vi "Signal property(SubVI).vi"(0 "Channel A":dbl[](array[numeric]), 1 "Analyze Channel":u16, 2 "DC level CH A":dbl, 3 "DC level CH B":dbl, 5 "Channel B":dbl[](array[numeric]), 7 "Channel A(FFT)":dbl[](array[numeric]), 9 "Channel B(FFT)":dbl[](array[numeric]), 11 "Frequency axis":dbl[](array[numeric]), 12 "Tones":enum32{"Single Tone", "Double tone", "Other"}(ring), 13 "Mark Signal Props":bool, 14 "Mark Harmonics":bool) -> (4 "Signal Property":string, 15 "Mark Signal Props":dbl[](array[numeric]))   [LabVIEW 2013]
uses:
  <vilib>/measure/matone.llb/SINAD Analyzer 1 Chan.vi
  <vilib>/measure/NI_MAPro.lvlib
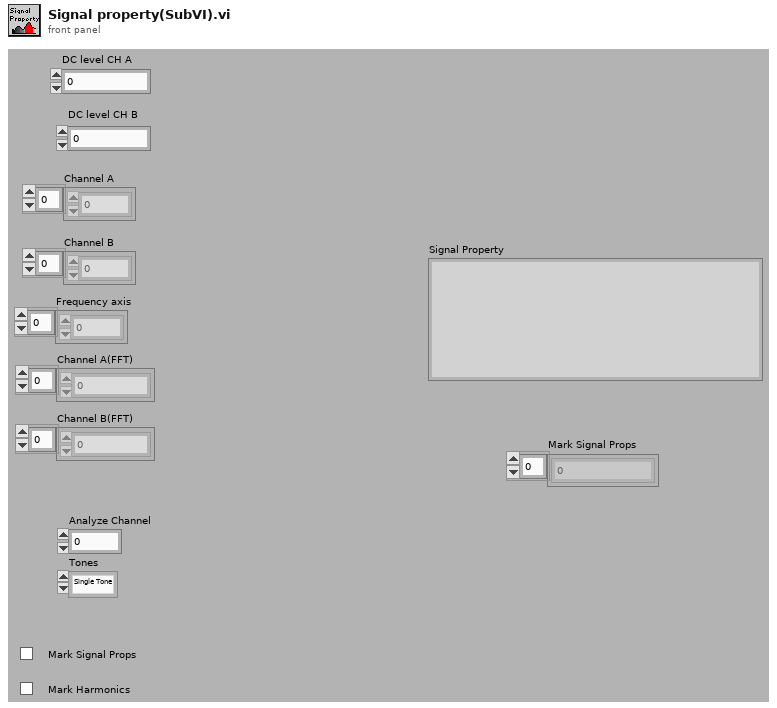
[diagram p1: front panel]
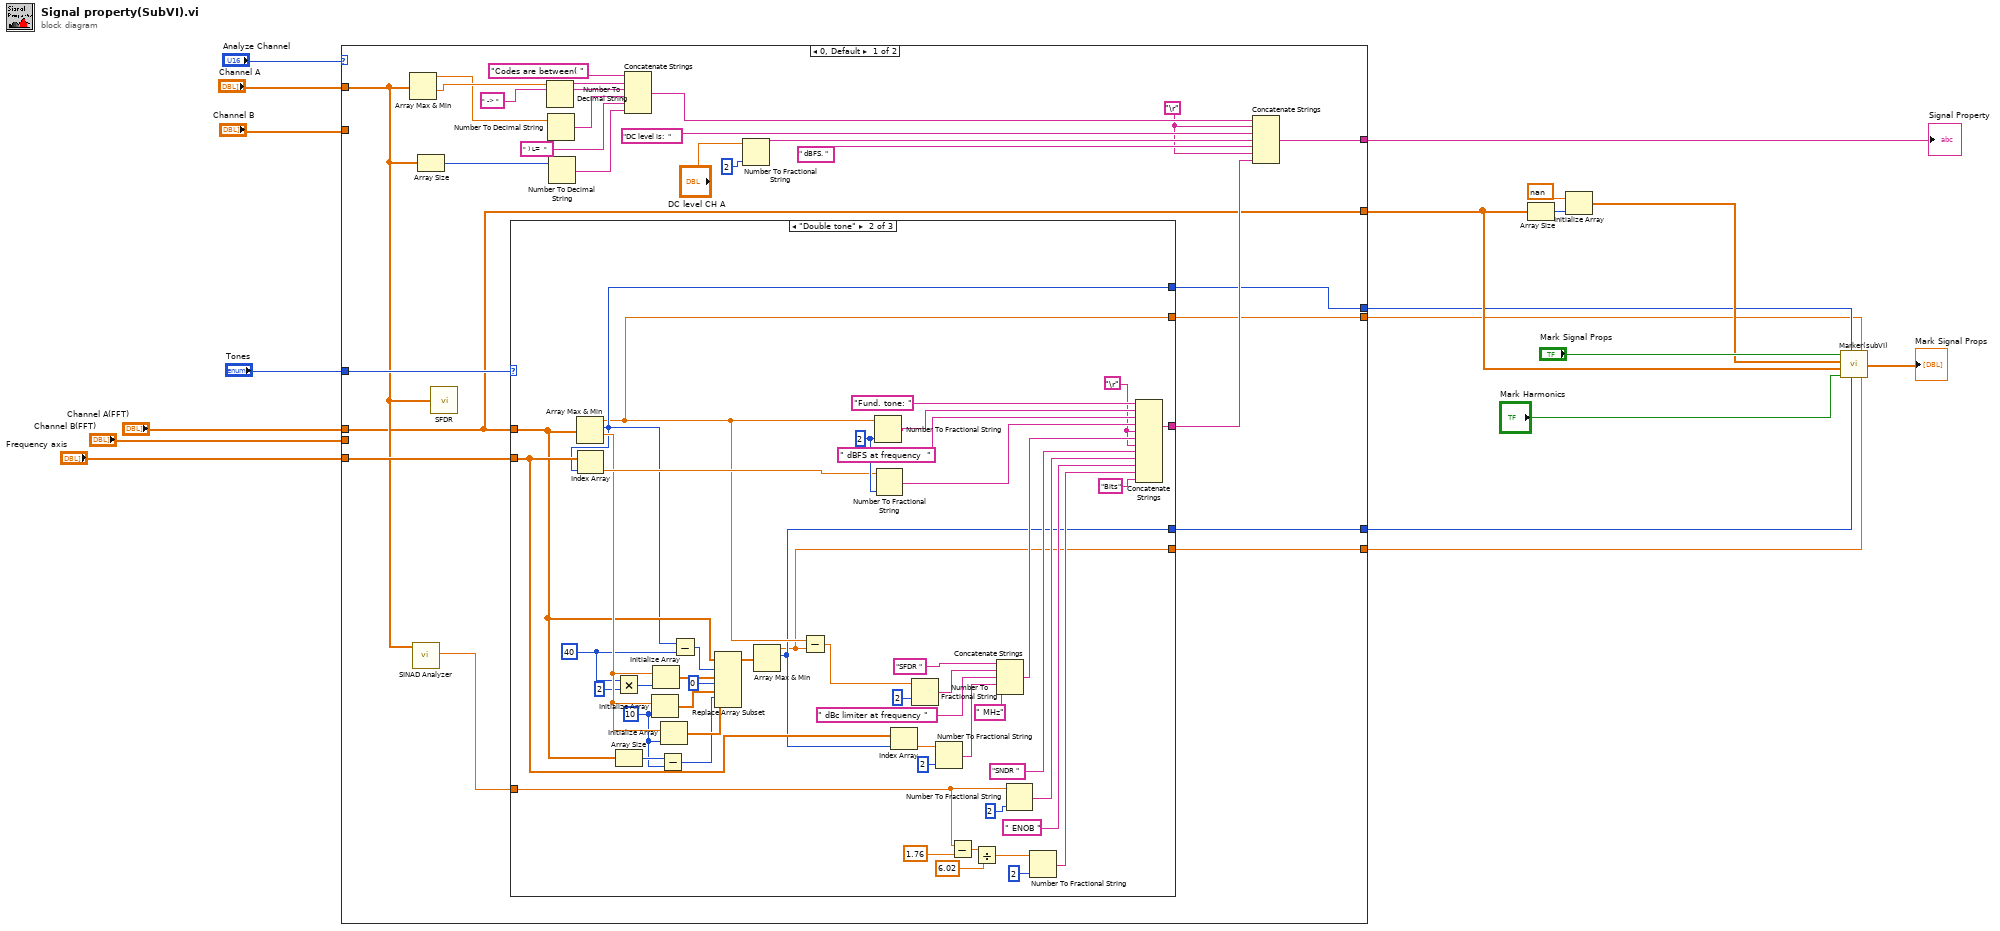
[diagram p0: block diagram]
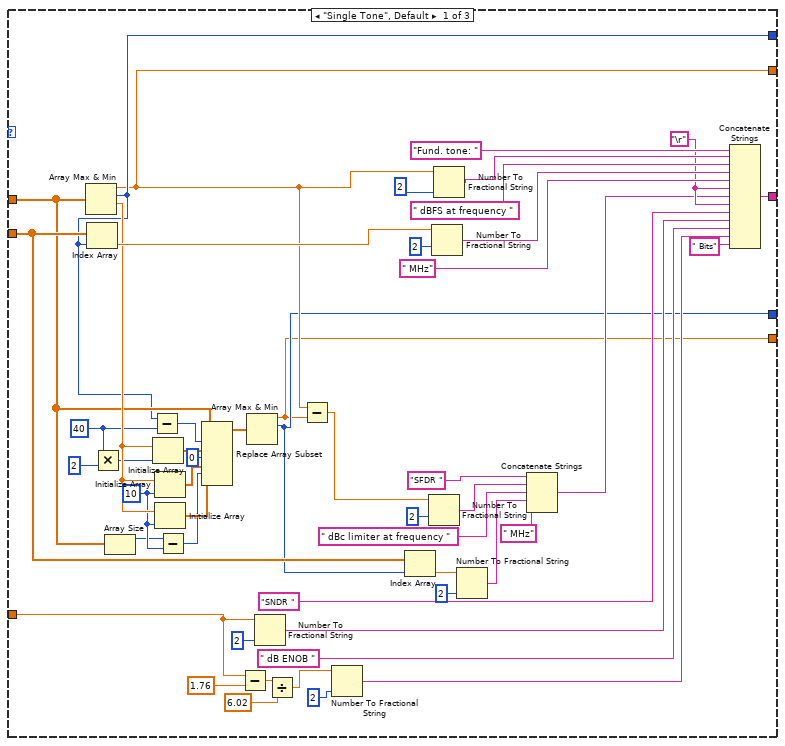
[diagram p2: hidden frame]
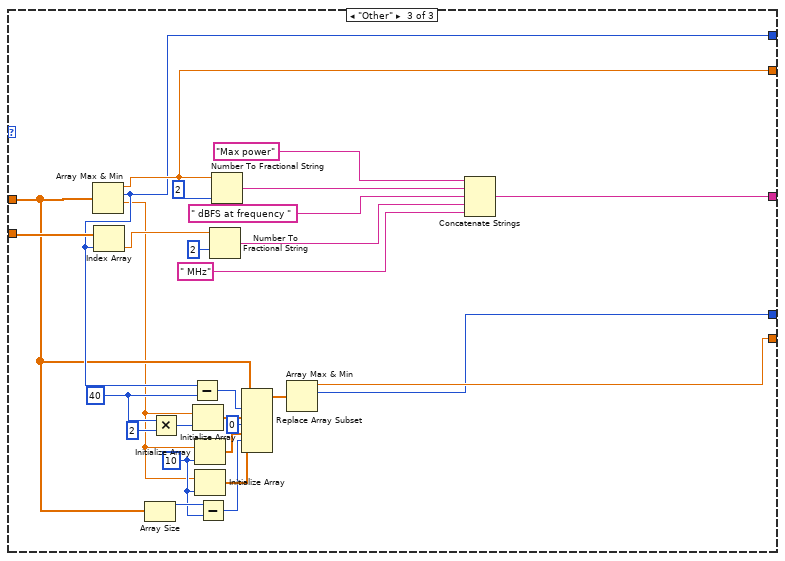
[diagram p3: hidden frame]
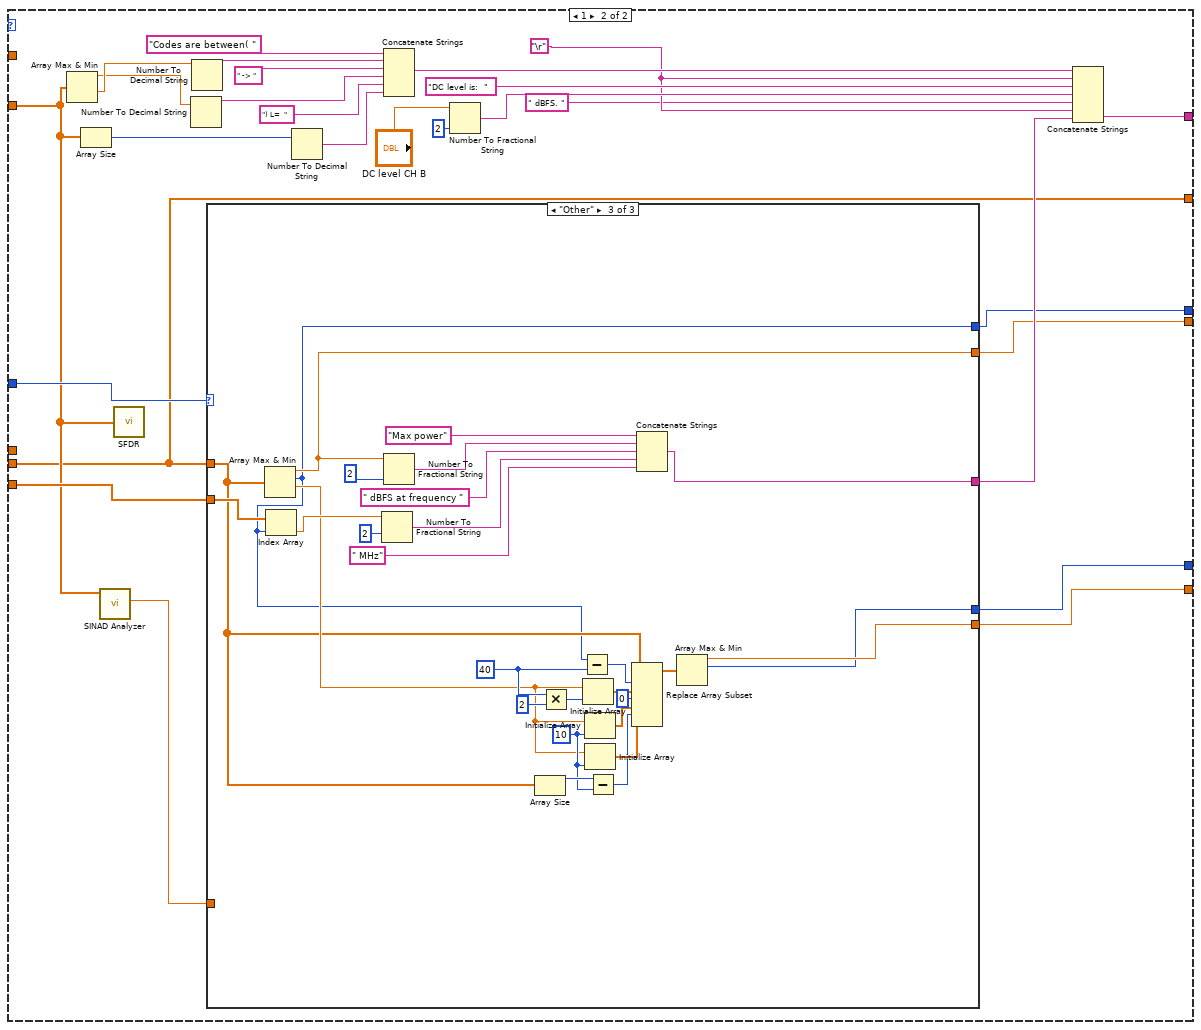
[diagram p4: hidden frame]
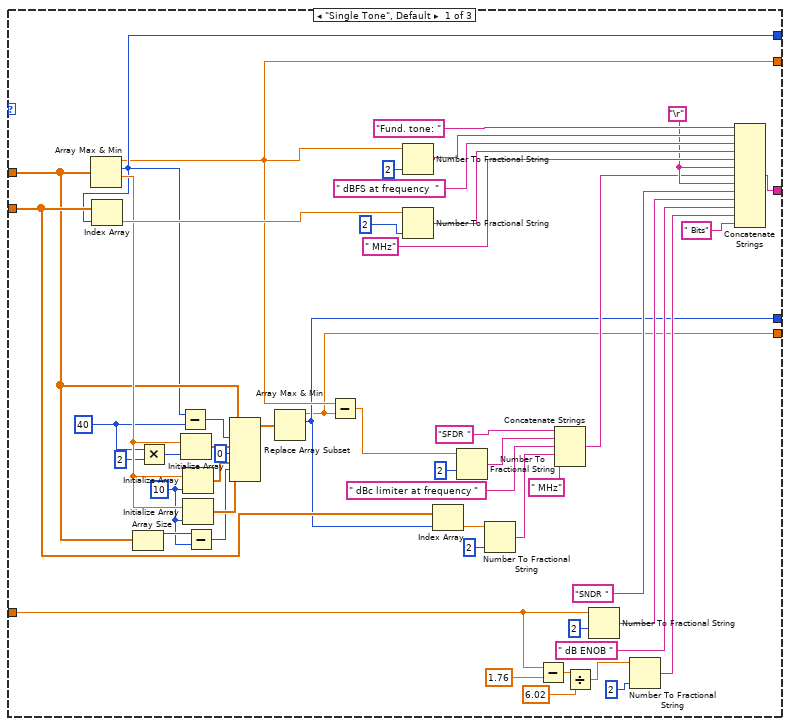
[diagram p5: hidden frame]
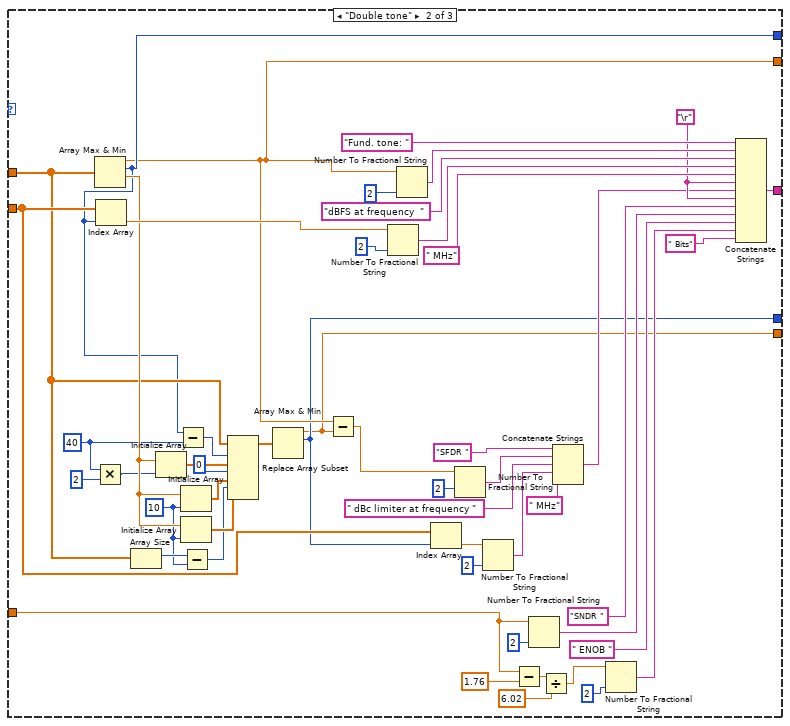
[diagram p6: hidden frame]
diagram:
  n1 = case shown="0, Default" "Analyze Channel" {
    tunnel: [w29 w197] -> w12
    tunnel: "Tones" -> [w40 w195]
    tunnel: "Channel A(FFT)" -> [w21 _]
    tunnel: "Channel B(FFT)" -> [_ w175]
    tunnel: "Frequency axis" -> [w35 w189]
    tunnel: "Channel B" -> [_ w181]
    tunnel: "Channel A" -> [w27 _]
    tunnel: [w24 w179] -> w5
    tunnel: [w23 w178] -> w4
    tunnel: [w20 w177] -> w3
    tunnel: [w22 w176] -> w2
    tunnel: [w21 w175] -> w6
    frame 0, Default {
      w31 = "\r"
      n2 = Array Max & Min(array=w27) -> (max value=w36:dbl, min value=w37:dbl)  [unwired: 2 out]
      n3 = call-poly <vilib>:"SINAD Analyzer.vi"("signal in"=w27) -> ("SINAD (dB)"=w28:dbl)  [unwired: 5 in, 5 out]
      n4 = Array Size(array=w27) -> (size(s)=w30:i32)
      n5 = call "SFDR.vi"("signal in"=w27) -> ()  [unwired: 1 out]
      n6 = case shown="\"Double tone\"" w40 {
        tunnel: [w94 w144 w173] -> w26
        tunnel: w21 -> [w51 w102 w150]
        tunnel: w35 -> [w59 w117 w169]
        tunnel: w28 -> [w77 w134 _]
        tunnel: [w50 w101 w151] -> w24
        tunnel: [w49 w100 w164] -> w23
        tunnel: [w48 w99 w147] -> w20
        tunnel: [w47 w98 w148] -> w22
        frame "Single Tone", Default {
          w57 = 10 ("dimension size")
          w54 = 40 ("y")
          w83 = "\r"
          n7 = Array Max & Min(array=w51) -> (max value=w49:dbl, max index (indices)=w50:i32, min value=w73:dbl)  [unwired: 1 out]
          n8 = Index Array(array=w59, index=w50) -> (element=w76:dbl)
          n9 = Multiply(x=w54, y=2) -> (x*y=w53:i32)
          n10 = Array Size(array=w51) -> (size(s)=w56:i32)
          n11 = Subtract(x=w50, y=w54) -> (x-y=w74:i32)
          n12 = Initialize Array(w73, w53) -> (w75:dbl[])
          n13 = Initialize Array(w73, w57) -> (w71:dbl[])
          n14 = Initialize Array(w73, w57) -> (w70:dbl[])
          n15 = Subtract(x=w56, y=w57) -> (x-y=w55:i32)
          n16 = Replace Array Subset(array=w51, new element #1=w75, index #1=w74, new element #2=w71, index #2=0 ("index"), new element #3=w70, index #3=w55) -> (w69:dbl[])
          n17 = Subtract(x=w77, y=1.76) -> (x-y=w88:dbl)
          n18 = Array Max & Min(array=w69) -> (max value=w47:dbl, max index (indices)=w48:i32)  [unwired: 2 out]
          n19 = Number To Fractional String(number=w77, precision (6)=i16 2) -> (F-format string=w81:string)  [unwired: 2 in]
          n20 = Divide(x=w88, y=6.02) -> (x/y=w85:dbl)
          n21 = Subtract(x=w49, y=w47) -> (x-y=w61:dbl)
          n22 = Number To Fractional String(number=w85, precision (6)=i16 2) -> (F-format string=w79:string)  [unwired: 2 in]
          n23 = Index Array(array=w59, index=w48) -> (element=w68:dbl)
          n24 = Number To Fractional String(number=w61, precision (6)=i16 2) -> (F-format string=w63:string)  [unwired: 2 in]
          n25 = Number To Fractional String(number=w76, precision (6)=i16 2) -> (F-format string=w93:string)  [unwired: 2 in]
          n26 = Number To Fractional String(number=w49, precision (6)=i16 2) -> (F-format string=w90:string)  [unwired: 2 in]
          n27 = Number To Fractional String(number=w68, precision (6)=i16 2) -> (F-format string=w66:string)  [unwired: 2 in]
          n28 = Concatenate Strings("SFDR ", w63, " dBc limiter at frequency ", w66, " MHz") -> (w58:string)
          n29 = Concatenate Strings("Fund. tone: ", w90, " dBFS at frequency ", w93, " MHz", w83, w58, w83, "SNDR ", w81, " dB ENOB ", w79, " Bits" ("string")) -> (w94:string)
        }
        frame "Double tone" {
          w107 = 10 ("dimension size")
          w104 = 40 ("y")
          w109 = "\r"
          w141 = i16 2 ("precision (6)")
          n30 = Array Max & Min(array=w102) -> (max value=w100:dbl, max index (indices)=w101:i32, min value=w116:dbl)  [unwired: 1 out]
          n31 = Index Array(array=w117, index=w101) -> (element=w133:dbl)
          n32 = Multiply(x=w104, y=2) -> (x*y=w105:i32)
          n33 = Array Size(array=w102) -> (size(s)=w108:i32)
          n34 = Initialize Array(w116, w107) -> (w129:dbl[])
          n35 = Initialize Array(w116, w105) -> (w132:dbl[])
          n36 = Subtract(x=w108, y=w107) -> (x-y=w106:i32)
          n37 = Initialize Array(w116, w107) -> (w128:dbl[])
          n38 = Subtract(x=w101, y=w104) -> (x-y=w131:i32)
          n39 = Replace Array Subset(array=w102, new element #1=w132, index #1=w131, new element #2=w129, index #2=0 ("index"), new element #3=w128, index #3=w106) -> (w127:dbl[])
          n40 = Array Max & Min(array=w127) -> (max value=w98:dbl, max index (indices)=w99:i32)  [unwired: 2 out]
          n41 = Subtract(x=w100, y=w98) -> (x-y=w119:dbl)
          n42 = Number To Fractional String(number=w100, precision (6)=w141) -> (F-format string=w142:string)  [unwired: 2 in]
          n43 = Number To Fractional String(number=w133, precision (6)=w141) -> (F-format string=w143:string)  [unwired: 2 in]
          n44 = Index Array(array=w117, index=w99) -> (element=w126:dbl)
          n45 = Number To Fractional String(number=w119, precision (6)=i16 2) -> (F-format string=w121:string)  [unwired: 2 in]
          n46 = Number To Fractional String(number=w126, precision (6)=i16 2) -> (F-format string=w124:string)  [unwired: 2 in]
          n47 = Subtract(x=w134, y=1.76) -> (x-y=w138:dbl)
          n48 = Divide(x=w138, y=6.02) -> (x/y=w135:dbl)
          n49 = Concatenate Strings("SFDR ", w121, " dBc limiter at frequency ", w124, " MHz") -> (w115:string)
          n50 = Number To Fractional String(number=w134, precision (6)=i16 2) -> (F-format string=w111:string)  [unwired: 2 in]
          n51 = Number To Fractional String(number=w135, precision (6)=i16 2) -> (F-format string=w113:string)  [unwired: 2 in]
          n52 = Concatenate Strings("Fund. tone: ", w142, " dBFS at frequency  ", w143, w109, w115, w109, "SNDR ", w111, " ENOB ", w113, "Bits" ("string")) -> (w144:string)
        }
        frame "Other" {
          w155 = 10 ("dimension size")
          w153 = 40 ("y")
          n53 = Array Max & Min(array=w150) -> (max value=w164:dbl, max index (indices)=w151:i32, min value=w149:dbl)  [unwired: 1 out]
          n54 = Index Array(array=w169, index=w151) -> (element=w170:dbl)
          n55 = Array Size(array=w150) -> (size(s)=w156:i32)
          n56 = Multiply(x=w153, y=2) -> (x*y=w154:i32)
          n57 = Subtract(x=w151, y=w153) -> (x-y=w162:i32)
          n58 = Initialize Array(w149, w154) -> (w163:dbl[])
          n59 = Initialize Array(w149, w155) -> (w160:dbl[])
          n60 = Initialize Array(w149, w155) -> (w159:dbl[])
          n61 = Subtract(x=w156, y=w155) -> (x-y=w157:i32)
          n62 = Number To Fractional String(number=w170, precision (6)=i16 2) -> (F-format string=w166:string)  [unwired: 2 in]
          n63 = Number To Fractional String(number=w164, precision (6)=i16 2) -> (F-format string=w168:string)  [unwired: 2 in]
          n64 = Replace Array Subset(array=w150, new element #1=w163, index #1=w162, new element #2=w160, index #2=0 ("index"), new element #3=w159, index #3=w157) -> (w158:dbl[])
          n65 = Array Max & Min(array=w158) -> (max value=w148:dbl, max index (indices)=w147:i32)  [unwired: 2 out]
          n66 = Concatenate Strings("Max power", w168, " dBFS at frequency ", w166, " MHz") -> (w173:string)
        }
      }
      n67 = Number To Decimal String(number=w37) -> (decimal integer string=w45:string)  [unwired: 1 in]
      n68 = Number To Decimal String(number=w36) -> (decimal integer string=w43:string)  [unwired: 1 in]
      n69 = Number To Decimal String(number=w30) -> (decimal integer string=w41:string)  [unwired: 1 in]
      n70 = Concatenate Strings("Codes are between( ", w45, " -> ", w43, " ) L=  ", w41) -> (w39:string)
      n71 = Number To Fractional String(number="DC level CH A", precision (6)=i16 2) -> (F-format string=w33:string)  [unwired: 2 in]
      n72 = Concatenate Strings(w39, w31, "DC level is:  ", w33, " dBFS. ", w31, w26) -> (w29:string)
    }
    frame 1 {
      w186 = "\r"
      n73 = Array Max & Min(array=w181) -> (max value=w187:dbl, min value=w188:dbl)  [unwired: 2 out]
      n74 = Array Size(array=w181) -> (size(s)=w183:i32)
      n75 = call-poly <vilib>:"SINAD Analyzer.vi"("signal in"=w181) -> ("SINAD (dB)"=w182:dbl)  [unwired: 5 in, 5 out]
      n76 = call "SFDR.vi"("signal in"=w181) -> ()  [unwired: 1 out]
      n77 = Number To Decimal String(number=w187) -> (decimal integer string=w192:string)  [unwired: 1 in]
      n78 = Number To Decimal String(number=w188) -> (decimal integer string=w193:string)  [unwired: 1 in]
      n79 = case shown="\"Other\"" w195 {
        tunnel: [w249 w300 w322] -> w185
        tunnel: w175 -> [w206 w257 w307]
        tunnel: w189 -> [w214 w267 w323]
        tunnel: w182 -> [w231 w282 _]
        tunnel: [w205 w256 w306] -> w179
        tunnel: [w204 w255 w321] -> w178
        tunnel: [w203 w254 w304] -> w177
        tunnel: [w202 w253 w305] -> w176
        frame "Single Tone", Default {
          w210 = 10 ("dimension size")
          w208 = 40 ("y")
          w237 = "\r"
          n80 = Array Max & Min(array=w206) -> (max value=w204:dbl, max index (indices)=w205:i32, min value=w215:dbl)  [unwired: 1 out]
          n81 = Index Array(array=w214, index=w205) -> (element=w244:dbl)
          n82 = Array Size(array=w206) -> (size(s)=w211:i32)
          n83 = Multiply(x=w208, y=2) -> (x*y=w209:i32)
          n84 = Subtract(x=w205, y=w208) -> (x-y=w229:i32)
          n85 = Initialize Array(w215, w209) -> (w230:dbl[])
          n86 = Initialize Array(w215, w210) -> (w227:dbl[])
          n87 = Initialize Array(w215, w210) -> (w226:dbl[])
          n88 = Subtract(x=w211, y=w210) -> (x-y=w212:i32)
          n89 = Replace Array Subset(array=w206, new element #1=w230, index #1=w229, new element #2=w227, index #2=0 ("index"), new element #3=w226, index #3=w212) -> (w225:dbl[])
          n90 = Array Max & Min(array=w225) -> (max value=w202:dbl, max index (indices)=w203:i32)  [unwired: 2 out]
          n91 = Subtract(x=w204, y=w202) -> (x-y=w217:dbl)
          n92 = Number To Fractional String(number=w204, precision (6)=i16 2) -> (F-format string=w248:string)  [unwired: 2 in]
          n93 = Number To Fractional String(number=w244, precision (6)=i16 2) -> (F-format string=w247:string)  [unwired: 2 in]
          n94 = Index Array(array=w214, index=w203) -> (element=w224:dbl)
          n95 = Number To Fractional String(number=w217, precision (6)=i16 2) -> (F-format string=w219:string)  [unwired: 2 in]
          n96 = Number To Fractional String(number=w224, precision (6)=i16 2) -> (F-format string=w222:string)  [unwired: 2 in]
          n97 = Subtract(x=w231, y=1.76) -> (x-y=w242:dbl)
          n98 = Concatenate Strings("SFDR ", w219, " dBc limiter at frequency ", w222, " MHz") -> (w213:string)
          n99 = Divide(x=w242, y=6.02) -> (x/y=w239:dbl)
          n100 = Number To Fractional String(number=w231, precision (6)=i16 2) -> (F-format string=w235:string)  [unwired: 2 in]
          n101 = Number To Fractional String(number=w239, precision (6)=i16 2) -> (F-format string=w233:string)  [unwired: 2 in]
          n102 = Concatenate Strings("Fund. tone: ", w248, " dBFS at frequency  ", w247, " MHz", w237, w213, w237, "SNDR ", w235, " dB ENOB ", w233, " Bits" ("string")) -> (w249:string)
        }
        frame "Double tone" {
          w262 = 10 ("dimension size")
          w260 = 40 ("y")
          w288 = "\r"
          n103 = Array Max & Min(array=w257) -> (max value=w255:dbl, max index (indices)=w256:i32, min value=w266:dbl)  [unwired: 1 out]
          n104 = Multiply(x=w260, y=2) -> (x*y=w259:i32)
          n105 = Index Array(array=w267, index=w256) -> (element=w295:dbl)
          n106 = Array Size(array=w257) -> (size(s)=w263:i32)
          n107 = Initialize Array(w266, w259) -> (w281:dbl[])
          n108 = Subtract(x=w256, y=w260) -> (x-y=w280:i32)
          n109 = Initialize Array(w266, w262) -> (w279:dbl[])
          n110 = Initialize Array(w266, w262) -> (w278:dbl[])
          n111 = Subtract(x=w263, y=w262) -> (x-y=w264:i32)
          n112 = Replace Array Subset(array=w257, new element #1=w281, index #1=w280, new element #2=w279, index #2=0 ("index"), new element #3=w278, index #3=w264) -> (w277:dbl[])
          n113 = Array Max & Min(array=w277) -> (max value=w253:dbl, max index (indices)=w254:i32)  [unwired: 2 out]
          n114 = Subtract(x=w255, y=w253) -> (x-y=w269:dbl)
          n115 = Number To Fractional String(number=w295, precision (6)=i16 2) -> (F-format string=w298:string)  [unwired: 2 in]
          n116 = Number To Fractional String(number=w255, precision (6)=i16 2) -> (F-format string=w299:string)  [unwired: 2 in]
          n117 = Index Array(array=w267, index=w254) -> (element=w276:dbl)
          n118 = Number To Fractional String(number=w269, precision (6)=i16 2) -> (F-format string=w271:string)  [unwired: 2 in]
          n119 = Number To Fractional String(number=w276, precision (6)=i16 2) -> (F-format string=w274:string)  [unwired: 2 in]
          n120 = Subtract(x=w282, y=1.76) -> (x-y=w293:dbl)
          n121 = Number To Fractional String(number=w282, precision (6)=i16 2) -> (F-format string=w286:string)  [unwired: 2 in]
          n122 = Divide(x=w293, y=6.02) -> (x/y=w290:dbl)
          n123 = Concatenate Strings("SFDR ", w271, " dBc limiter at frequency ", w274, " MHz") -> (w265:string)
          n124 = Number To Fractional String(number=w290, precision (6)=i16 2) -> (F-format string=w285:string)  [unwired: 2 in]
          n125 = Concatenate Strings("Fund. tone: ", w299, "dBFS at frequency  ", w298, " MHz", w288, w265, w288, "SNDR ", w286, " ENOB ", w285, " Bits" ("string")) -> (w300:string)
        }
        frame "Other" {
          w312 = 10 ("dimension size")
          w310 = 40 ("y")
          n126 = Array Max & Min(array=w307) -> (max value=w321:dbl, max index (indices)=w306:i32, min value=w308:dbl)  [unwired: 1 out]
          n127 = Index Array(array=w323, index=w306) -> (element=w328:dbl)
          n128 = Number To Fractional String(number=w328, precision (6)=i16 2) -> (F-format string=w325:string)  [unwired: 2 in]
          n129 = Number To Fractional String(number=w321, precision (6)=i16 2) -> (F-format string=w327:string)  [unwired: 2 in]
          n130 = Array Size(array=w307) -> (size(s)=w313:i32)
          n131 = Multiply(x=w310, y=2) -> (x*y=w311:i32)
          n132 = Subtract(x=w306, y=w310) -> (x-y=w319:i32)
          n133 = Initialize Array(w308, w311) -> (w320:dbl[])
          n134 = Initialize Array(w308, w312) -> (w317:dbl[])
          n135 = Initialize Array(w308, w312) -> (w316:dbl[])
          n136 = Subtract(x=w313, y=w312) -> (x-y=w314:i32)
          n137 = Replace Array Subset(array=w307, new element #1=w320, index #1=w319, new element #2=w317, index #2=0 ("index"), new element #3=w316, index #3=w314) -> (w315:dbl[])
          n138 = Concatenate Strings("Max power", w327, " dBFS at frequency ", w325, " MHz") -> (w322:string)
          n139 = Array Max & Min(array=w315) -> (max value=w305:dbl, max index (indices)=w304:i32)  [unwired: 2 out]
        }
      }
      n140 = Number To Decimal String(number=w183) -> (decimal integer string=w191:string)  [unwired: 1 in]
      n141 = Concatenate Strings("Codes are between( ", w193, " -> ", w192, ") L=  ", w191) -> (w196:string)
      n142 = Number To Fractional String(number="DC level CH B", precision (6)=i16 2) -> (F-format string=w194:string)  [unwired: 2 in]
      n143 = Concatenate Strings(w196, w186, "DC level is:  ", w194, " dBFS. ", w186, w185) -> (w197:string)
    }
  }
  "Signal Property" <- w12
  n144 = Array Size(array=w6) -> (size(s)=w11:i32)
  n145 = Initialize Array(nan ("element"), w11) -> (w7:dbl[])
  n146 = call "Marker(subVI).vi"("Mark Signal Props"="Mark Signal Props", "Fund indx"=w5, "Marki signal"=w7, "FFT"=w6, "SFDR indx"=w3, "Mark Harmonics"="Mark Harmonics", "Fund value"=w4, "SFDR VALUE"=w2) -> ("Output marking"=→"Mark Signal Props":dbl[])
